vi "표지판 인식 횟수 이벤트 발생.vi"() -> ()   [LabVIEW 2016]
panel:
  out "ms 타이머 값":u32
  in  "정적 횟수":u8
  in  "유턴 횟수":u8
  in  "동적 횟수":u8
  in  "주차냐 3":bool
  in  "주차냐 2":bool
  in  "주차냐":bool
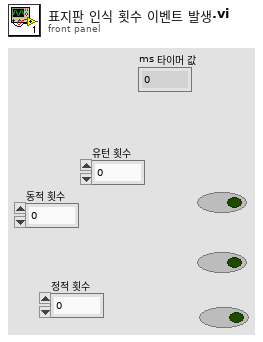
[diagram p1: front panel]
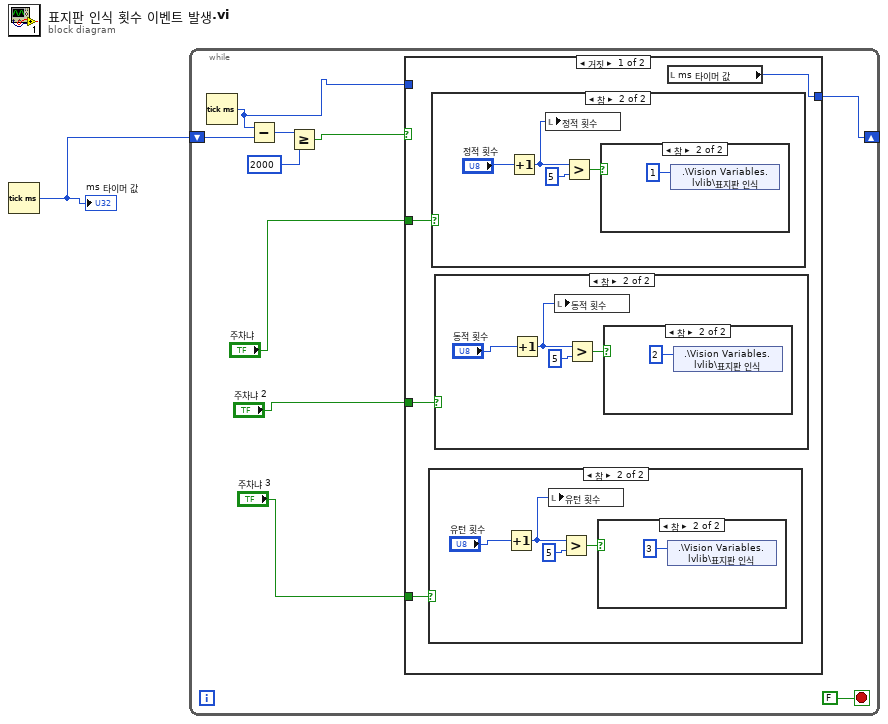
[diagram p0: block diagram]
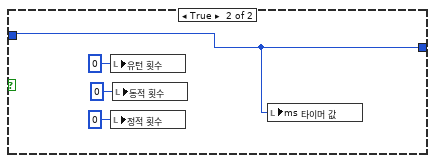
[diagram p8: hidden frame]
diagram:
  n1 = Tick Count (ms)() -> (millisecond timer value=w1:u32)
  "ms 타이머 값" <- w1
  n2 = while {
    shift-right: [w2] -> _
    shift-left: w1 -> [w11]
    stop <- FALSE stop-if-true
    n3 = Tick Count (ms)() -> (millisecond timer value=w3:u32)
    n4 = Subtract(x=w3, y=w11) -> (x-y=w10:u32)
    n5 = Greater Or Equal?(x=w10, y=u32 2000) -> (x >= y?=w7:bool)
    n6 = case shown="거짓" w7 {
      tunnel: "주차냐" -> [w15 _]
      tunnel: "주차냐 2" -> [w14 _]
      tunnel: "주차냐 3" -> [w13 _]
      tunnel: w3 -> [_ w31]
      tunnel: [w12 w31] -> w2
      frame False {
        n7 = case shown="참" w13 {
          frame False {
          }
          frame True {
            n8 = Increment(x="유턴 횟수") -> (x+1=w17:u8)
            n9 = local write "유턴 횟수"(w17) -> ()
            n10 = Greater?(x=w17, y=u8 5) -> (0:w18:bool)
            n11 = case shown="참" w18 {
              frame False {
              }
              frame True {
                n12 = shared-variable ".\\Vision Variables.lvlib\\표지판 인식"(u8 3 ("표지판 인식")) -> ()  [unwired: 1 in, 1 out]
              }
            }
          }
        }
        n13 = case shown="참" w15 {
          frame False {
          }
          frame True {
            n14 = Increment(x="정적 횟수") -> (x+1=w28:u8)
            n15 = local write "정적 횟수"(w28) -> ()
            n16 = Greater?(x=w28, y=u8 5) -> (0:w27:bool)
            n17 = case shown="참" w27 {
              frame False {
              }
              frame True {
                n18 = shared-variable ".\\Vision Variables.lvlib\\표지판 인식"(u8 1 ("표지판 인식")) -> ()  [unwired: 1 in, 1 out]
              }
            }
          }
        }
        n19 = case shown="참" w14 {
          frame False {
          }
          frame True {
            n20 = Increment(x="동적 횟수") -> (x+1=w21:u8)
            n21 = local write "동적 횟수"(w21) -> ()
            n22 = Greater?(x=w21, y=u8 5) -> (0:w23:bool)
            n23 = case shown="참" w23 {
              frame False {
              }
              frame True {
                n24 = shared-variable ".\\Vision Variables.lvlib\\표지판 인식"(u8 2 ("표지판 인식")) -> ()  [unwired: 1 in, 1 out]
              }
            }
          }
        }
        n25 = local read "ms 타이머 값"() -> (w12:u32)
      }
      frame True {
        n26 = local write "유턴 횟수"(u8 0 ("유턴 횟수")) -> ()
        n27 = local write "정적 횟수"(u8 0 ("유턴 횟수")) -> ()
        n28 = local write "동적 횟수"(u8 0 ("유턴 횟수")) -> ()
        n29 = local write "ms 타이머 값"(w31) -> ()
      }
    }
  }
